vi "Target 2 Record.vi"(8 "Active Matrices":T1[](array[typedef]), 9 "Step":string, 10 "Current Target In":T2[](array[typedef]), 11 "Time Stamp":timestamp) -> (2 "String Records Out":string[](array[string]))   [LabVIEW 2009]
uses:
  MixedMode/Target Data.ctl
  Archive File Type.ctl
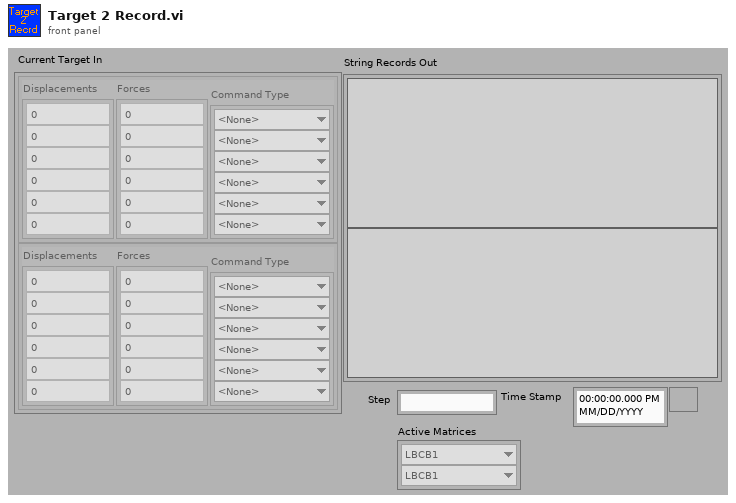
[diagram p1: front panel]
types:
  T1 = typedef "Archive File Type.ctl" = enum16{"LBCB1", "LBCB2", "ExternalSensors", "Combined"}
  T2 = typedef "Target Data.ctl" = cluster{"Displacements":dbl[], "Command Type":enum16{"<None>", "Displacement", "Force"}[], "Forces":dbl[]}
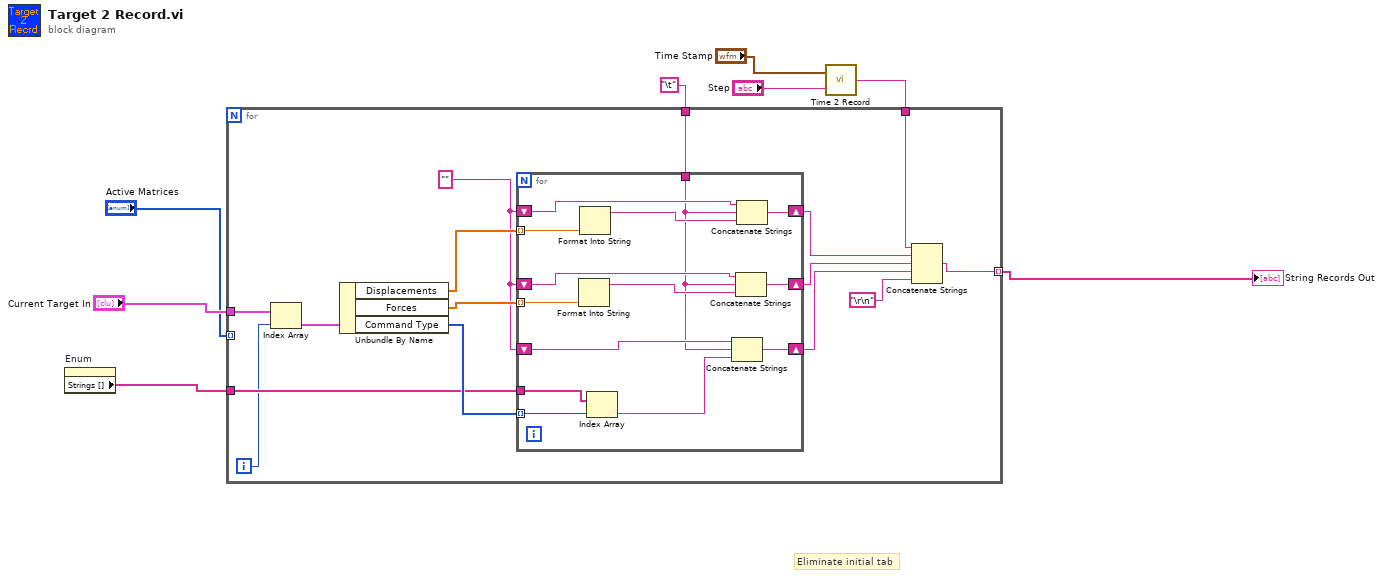
[diagram p0: block diagram]
diagram:
  # "Eliminate initial tab"
  n1 = property on="Enum" class="Enum (strict)"() -> ("Strings []"=w7:string[])  [unwired: 2 in, 2 out]
  n2 = call "Time 2 Record.vi"("Step"="Step", "Time Stamp"="Time Stamp") -> ("String"=w5:string)
  n3 = for {
    tunnel: "Current Target In" -> [w23]
    tunnel: w7 -> [w19]
    tunnel: "\t" -> [w18]
    tunnel: [w17] -> w1 mode=indexing
    tunnel: w5 -> [w13]
    tunnel: "Active Matrices" -> [_] mode=indexing
    i -> [w9]
    w12 = ""
    n4 = Index Array(array=w23, index=w9) -> (element=w10:T2)
    n5 = Unbundle By Name(w10) -> ("Displacements"=w22:dbl[], "Forces"=w21:dbl[], "Command Type"=w20:enum16{"<None>", "Displacement", "Force"}[])
    n6 = for {
      tunnel: w22 -> [w37] mode=indexing
      tunnel: w21 -> [w36] mode=indexing
      tunnel: w20 -> [w35] mode=indexing
      tunnel: w19 -> [w34]
      shift-right: [w26] -> w16
      shift-left: w12 -> [w30]
      shift-right: [w25] -> w15
      shift-left: w12 -> [w29]
      shift-right: [w24] -> w14
      shift-left: w12 -> [w28]
      tunnel: w18 -> [w27]
      n7 = Format Into String(w36) -> (resulting string=w32:string)  [unwired: 3 in, 1 out]
      n8 = Format Into String(w37) -> (resulting string=w33:string)  [unwired: 3 in, 1 out]
      n9 = Index Array(array=w34, index=w35) -> (element=w31:string)
      n10 = Concatenate Strings(w28, w27, w31) -> (w24:string)
      n11 = Concatenate Strings(w29, w27, w32) -> (w25:string)
      n12 = Concatenate Strings(w30, w27, w33) -> (w26:string)
    }
    n13 = Concatenate Strings(w13, w16, w15, w14, "\r\n") -> (w17:string)
  }
  "String Records Out" <- w1
